vi "scan injector.vi"() -> ()   [LabVIEW 2016]
uses:
  <vilib>/Utility/file.llb/Write Delimited Spreadsheet (DBL).vi
  Top level/Top Level.lvlib
  <vilib>/Analysis/NI_AALPro.lvlib
panel:
  out "Slide":dbl(slide) scale=0.0..10.0
  out "data":dbl
  out "x+y":dbl
  out "x+1":dbl
  out "error out":errorcluster
  out "# found":i32
  out "current":dbl[](graph)
  out "step size":dbl
  in  "time wait(sec)":dbl=2.0
  in  "number of steps":dbl=500.0
  in  "end value":dbl=1.0
  in  "start value":dbl
  in  "OK Button":bool
  in  "stop":bool
  # "set injector field to start value before beginning.  \nonce done,  a dialog box will pop up and ask where\nthe file should be stored."
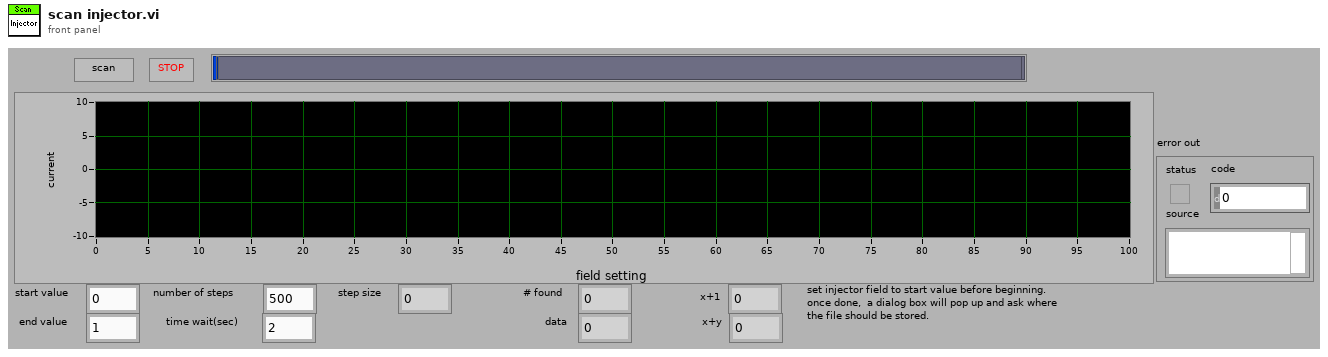
[diagram p1: front panel]
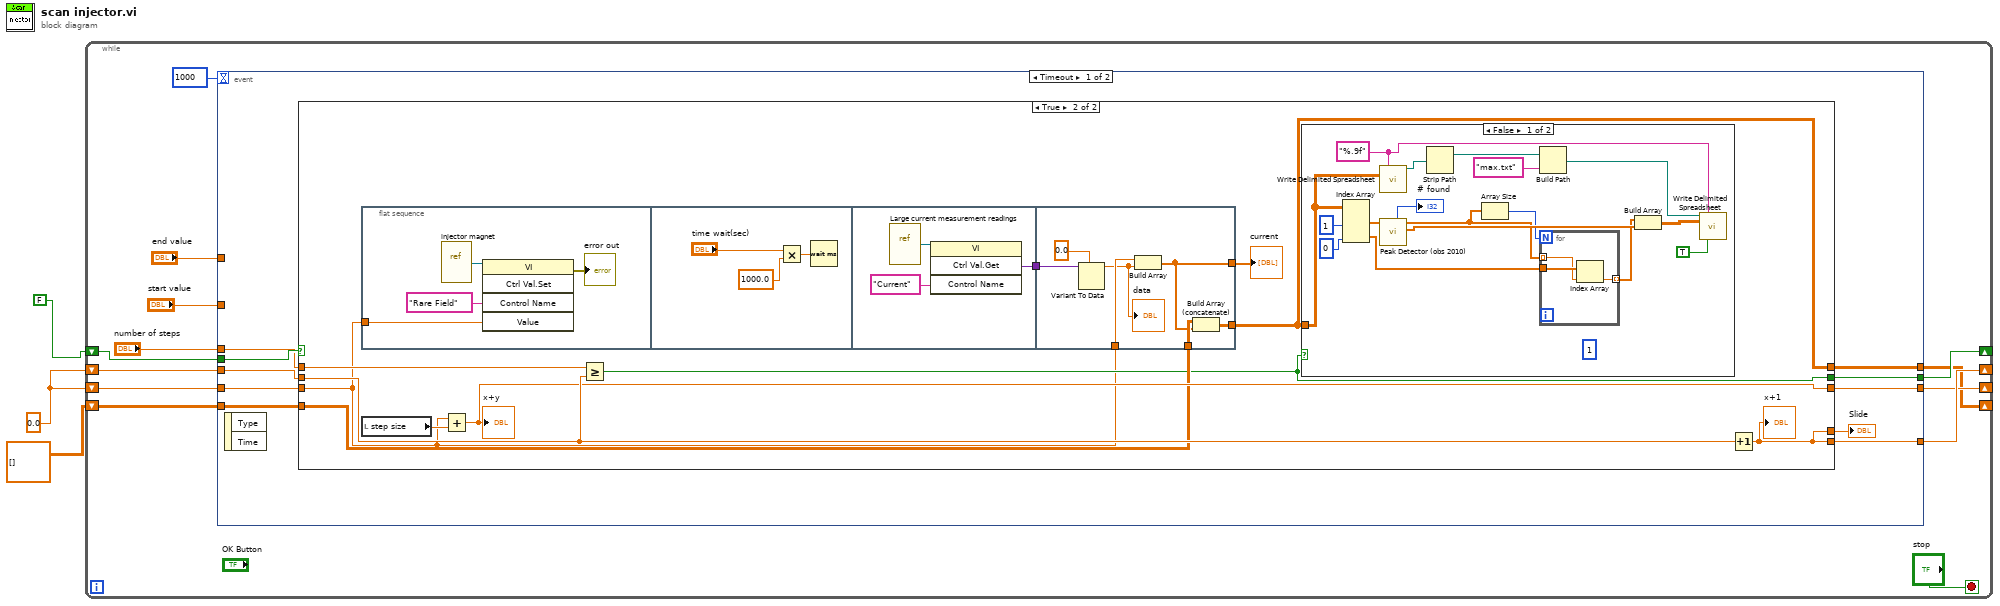
[diagram p0: block diagram]
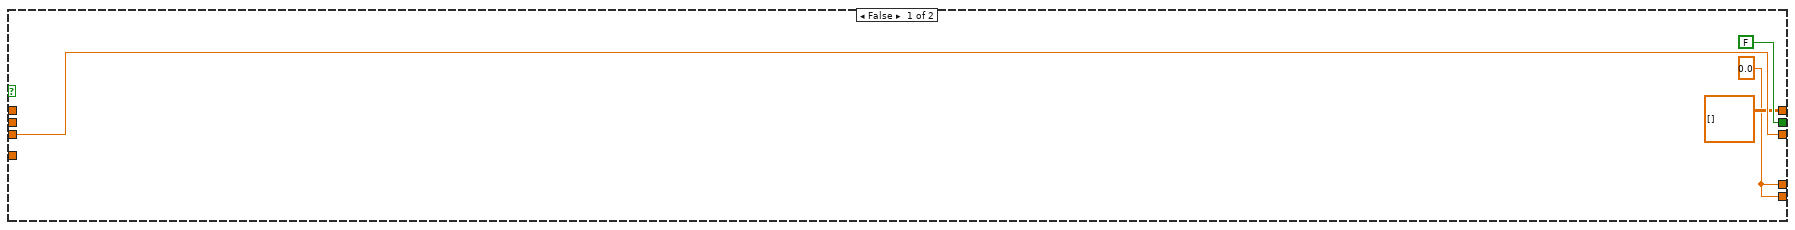
[diagram p2: hidden frame]
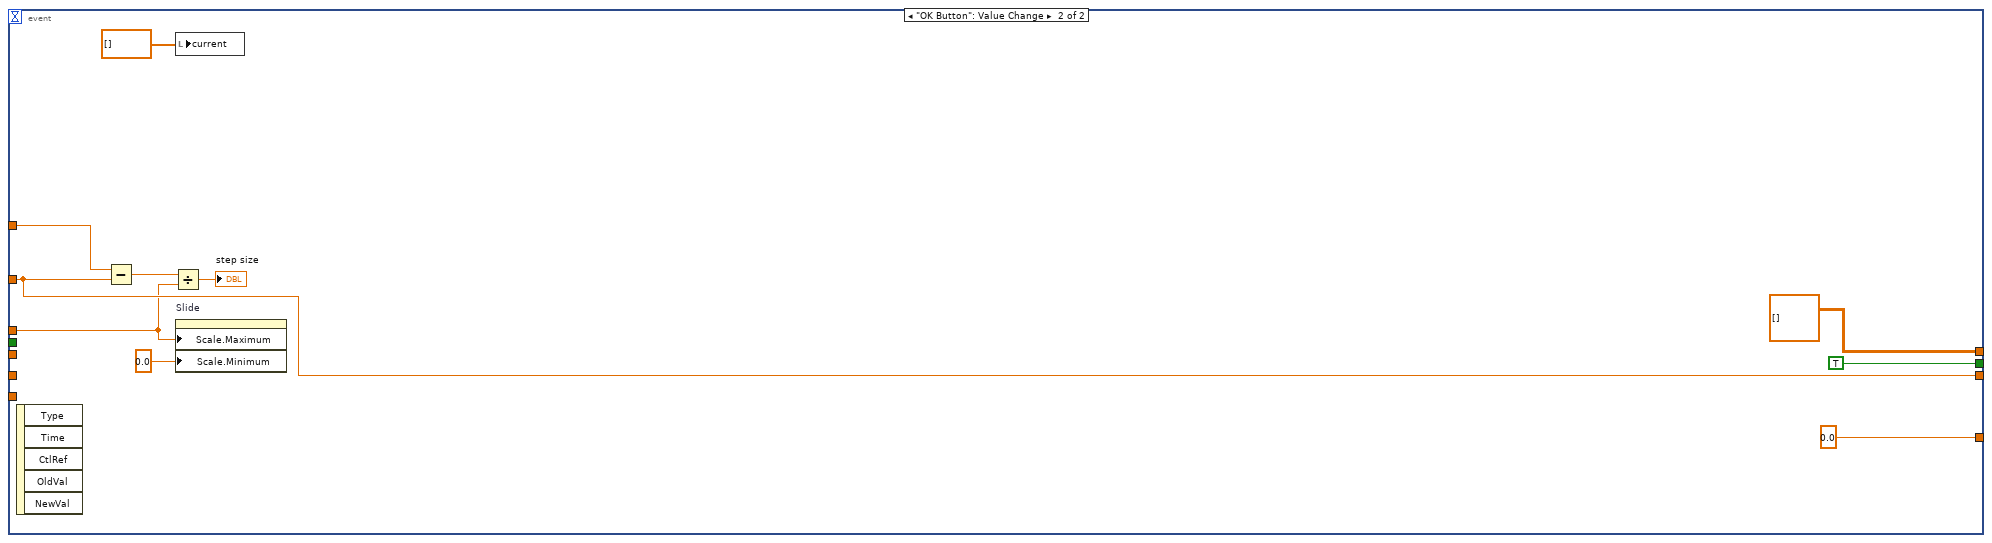
[diagram p4: hidden frame]
diagram:
  w2 = 0.0 ("number of steps")
  n1 = while {
    shift-right: [w14] -> _
    shift-left: FALSE -> [w15]
    shift-right: [w13] -> _
    shift-left: w2 -> [w12]
    shift-right: [w8] -> _
    shift-left: w2 -> [w4]
    shift-right: [w5] -> _
    shift-left: dbl[][] [] -> [w6]
    stop <- "stop" stop-if-true
    n2 = event shown="[0] Timeout" {
      selector: _ -> [_ _]
      dyn-events: _ -> [_ _]
      timeout: 1000 -> [_ _]
      tunnel: w15 -> [w26 _]
      tunnel: [w25 TRUE] -> w14
      tunnel: [w24 0.0 ("number of steps")] -> w13
      tunnel: w12 -> [w23 _]
      tunnel: "start value" -> [_ w81]
      tunnel: "end value" -> [_ w82]
      tunnel: "number of steps" -> [w22 w79]
      tunnel: [w21 w81] -> w8
      tunnel: [w20 dbl[][] []] -> w5
      tunnel: w6 -> [w19 _]
      tunnel: w4 -> [w18 _]
      event Timeout {
        n3 = event-data() -> ()  [unwired: 1 in, 2 out]
        n4 = case shown="True" w26 {
          tunnel: [FALSE w35] -> w25
          tunnel: [w27 w31] -> w24
          tunnel: w23 -> [_ w41]
          tunnel: w22 -> [_ w40]
          tunnel: [w29 w39] -> w21
          tunnel: w18 -> [w29 w33]
          tunnel: [dbl[][] [] w34] -> w20
          tunnel: w19 -> [_ w36]
          tunnel: [w27 w31] -> w17
          frame False {
            w27 = 0.0 ("number of steps")
          }
          frame True {
            n5 = flat-sequence {
              tunnel: w33 -> [w63]
              tunnel: [w69] -> w38
              tunnel: w38 -> [w78]
              tunnel: w33 -> [w76]
              tunnel: [w73] -> w32
              tunnel: w36 -> [w74]
              tunnel: [w72] -> w34
              frame #0 {
                n6 = vi-ref "injector magnet.vi"() -> (w65:refnum<vi>)
                n7 = invoke class="VI" method="Ctrl Val.Set"(reference=w65, "Control Name"="Rare Field", "Value"=w63) -> (error out=→"error out":errorcluster)  [unwired: 2 in, 4 out]
              }
              frame #1 {
                n8 = Multiply(x="time wait(sec)", y=1000.0) -> (x*y=w66:dbl)
                n9 = Wait (ms)(milliseconds to wait=w66) -> ()  [unwired: 1 out]
              }
              frame #2 {
                n10 = vi-ref "Large current measurement readings.vi"() -> (w71:refnum<vi>)
                n11 = invoke class="VI" method="Ctrl Val.Get"(reference=w71, "Control Name"="Current") -> ("Get Control Value Variant"=w69:variant)  [unwired: 2 in, 3 out]
              }
              frame #3 {
                n12 = Variant To Data(type=0.0 ("y"), Variant=w78) -> (data=w75:dbl)  [unwired: 1 in, 1 out]
                "data" <- w75
                n13 = Build Array(w76, w75) -> (w73:dbl[])
                n14 = Build Array (concatenate)(w74, w73) -> (w72:dbl[][])
              }
            }
            n15 = local read "step size"() -> (w37:dbl)
            n16 = Add(x=w33, y=w37) -> (x+y=w39:dbl)
            "x+y" <- w39
            n17 = Greater Or Equal?(x=w40, y=w41) -> (x >= y?=w35:bool)
            n18 = case shown="False" w35 {
              tunnel: w34 -> [w54 _]
              frame False {
                w43 = "%.9f" ("format (%.3f)")
                (unwired) 1 ("width")
                n19 = Index Array(array=w54, index (col) #1=1 ("index"), index (col) #2=0 ("index (col)")) -> (element #1=w57:dbl[], element #2=w46:dbl[])  [unwired: 2 in]
                n20 = call-poly <vilib>:"Write Delimited Spreadsheet.vi"("format (%.3f)"=w43, "2D data"=w54) -> ("new file path (Not A Path if cancelled)"=w53:path)  [unwired: 12 in, 1 out]
                n21 = call <vilib>:"Peak Detector (obs 2010).vi"("X"=w57) -> ("Amplitudes"=w55:dbl[], "Locations"=w48:dbl[], "# found"=→"# found":i32)  [unwired: 6 in, 2 out]
                n22 = Strip Path(path=w53) -> (stripped path=w52:path)  [unwired: 1 out]
                n23 = Array Size(array=w48) -> (size(s)=w47:i32)
                n24 = Build Path(base path=w52, name or relative path="max.txt") -> (appended path=w50:path)
                n25 = for {
                  N: w47 -> [_]
                  tunnel: w48 -> [w60] mode=indexing
                  tunnel: w46 -> [w61]
                  tunnel: [w59] -> w44 mode=indexing
                  n26 = Index Array(array=w61, index=w60) -> (element=w59:dbl)
                }
                n27 = Build Array(w44, w55) -> (w45:dbl[][])
                n28 = call-poly <vilib>:"Write Delimited Spreadsheet.vi"("file path (dialog if empty)"=w50, "format (%.3f)"=w43, "2D data"=w45, "transpose? (no:F)"=TRUE) -> ()  [unwired: 10 in, 2 out]
              }
              frame True {
              }
            }
            n29 = Increment(x=w41) -> (x+1=w31:dbl)
            "x+1" <- w31
            "current" <- w32
          }
        }
        "Slide" <- w17
      }
      event "OK Button": Value Change {
        n30 = event-data() -> ()  [unwired: 1 in, 5 out]
        n31 = Subtract(x=w82, y=w81) -> (x-y=w83:dbl)
        n32 = Divide(x=w83, y=w79) -> (x/y=→"step size":dbl)
        n33 = local write "current"(dbl[] []) -> ()
        n34 = property on="Slide" class="Slide (strict)"("Scale.Maximum"=w79, "Scale.Minimum"=0.0 ("Scale.Range:Minimum")) -> ()  [unwired: 2 in, 2 out]
      }
    }
  }
